vi "Scaling (Sensitivity).vi"(0 "waveforms in":waveform(dbl)[](array[waveform]), 5 "sensitivity":dbl[](array[numeric]), 9 "system info in":refnum<class "EP System Info.lvclass">, 11 "error in (no error)":errorcluster) -> (4 "waveforms out":waveform(dbl)[](array[waveform]), 10 "system info out":refnum<class "EP System Info.lvclass">, 15 "error out":errorcluster)   [LabVIEW 2014, in "NI_EP_Power Quality.lvlib"]
doc: "Scales waveforms based on the sensitivity of the voltage/current transformer or transducer. You must manually select the polymorphic instance you want to use.\n\nThis VI supports measuring single-line and multiple-line systems."
uses:
  <vilib>/addons/Electrical Power/PQ/NI_EP_Power Quality.lvlib
  <vilib>/addons/Electrical Power/PQ/Common/Classes/System Info/EP System Info.lvclass
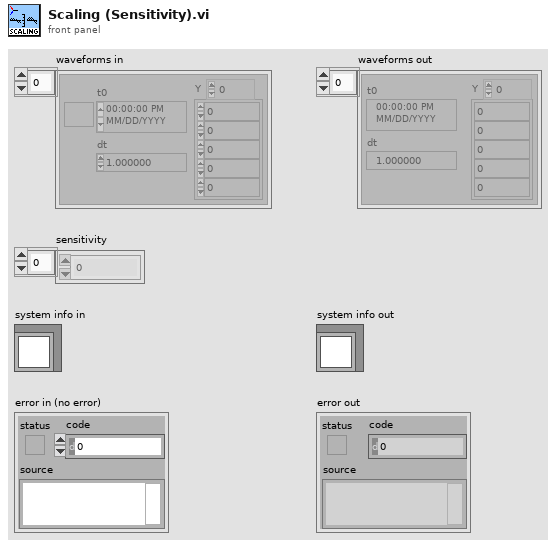
[diagram p1: front panel]
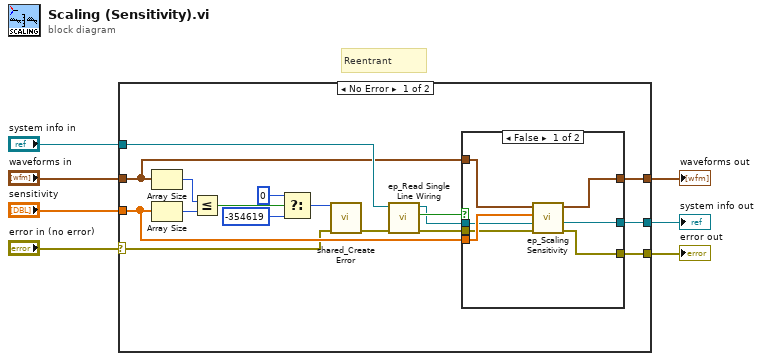
[diagram p0: block diagram]
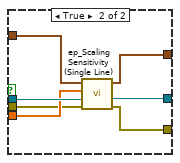
[diagram p2: hidden frame]
diagram:
  # "Reentrant"
  n1 = case shown="No Error" "error in (no error)" {
    selector: "error in (no error)" -> [w8 w39]
    tunnel: "system info in" -> [w18 w40]
    tunnel: "sensitivity" -> [w14 _]
    tunnel: "waveforms in" -> [w13 w41]
    tunnel: [w11 w41] -> w4
    tunnel: [w10 w40] -> w3
    tunnel: [w9 w39] -> w2
    frame No Error {
      n2 = Array Size(array=w13) -> (size(s)=w23:i32)
      n3 = Array Size(array=w14) -> (size(s)=w24:i32)
      n4 = Less Or Equal?(x=w23, y=w24) -> (x <= y?=w22:bool)
      n5 = Select(t=0 ("error code (0)"), s=w22, f=-354619 ("error code (0)")) -> (s? t:f=w19:i32)
      n6 = call <vilib>:"shared_Create Error.vi"("error in (no error)"=w8, "error code (0)"=w19) -> ("error out"=w17:errorcluster)  [unwired: 9 in]
      n7 = call <vilib>:"ep_Read Single Line Wiring.vi"("error in (no error)"=w17, "system info in"=w18) -> ("error out"=w12:errorcluster, "single line wiring? (F)"=w16:bool, "system info out"=w15:refnum<class "EP System Info.lvclass">)  [unwired: 7 in]
      n8 = case shown="False" w16 {
        tunnel: w15 -> [w29 w38]
        tunnel: w14 -> [w30 w37]
        tunnel: w13 -> [w31 w36]
        tunnel: w12 -> [w28 w35]
        tunnel: [w27 w34] -> w11
        tunnel: [w26 w33] -> w10
        tunnel: [w25 w32] -> w9
        frame False {
          n9 = call <vilib>:"ep_Scaling Sensitivity.vi"("error in (no error)"=w28, "system info in"=w29, "sensitivity"=w30, "waveforms in"=w31) -> ("error out"=w25:errorcluster, "system info out"=w26:refnum<class "EP System Info.lvclass">, "waveforms out"=w27:waveform(dbl)[])  [unwired: 5 in]
        }
        frame True {
          n10 = call <vilib>:"ep_Scaling Sensitivity (Single Line).vi"("error in (no error)"=w35, "system info in"=w38, "sensitivity"=w37, "waveforms in"=w36) -> ("error out"=w32:errorcluster, "system info out"=w33:refnum<class "EP System Info.lvclass">, "waveforms out"=w34:waveform(dbl)[])  [unwired: 5 in]
        }
      }
    }
    frame Error {
    }
  }
  "waveforms out" <- w4
  "error out" <- w2
  "system info out" <- w3
